vi "Select.vi"(0 "Father":u8[](array[numeric]) format="0x%02x", 2 "Mother":u8[](array[numeric]) format="0x%02x", 3 "Target":u8[](array[numeric]) format="0x%02x") -> (1 "Runnerup":u8[](array[numeric]) format="0x%02x", 4 "Winner":u8[](array[numeric]) format="0x%02x")   [LabVIEW 2013]
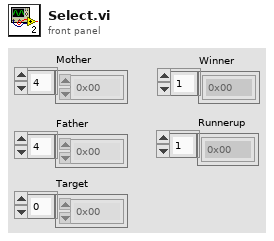
[diagram p1: front panel]
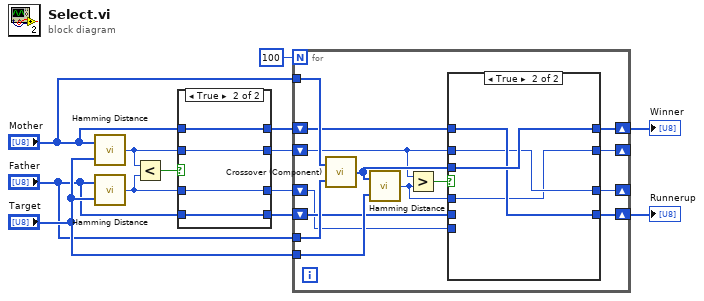
[diagram p0: block diagram]
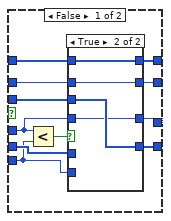
[diagram p2: hidden frame]
diagram:
  n1 = call "Hamming Distance.vi"("LED 2"="Target", "LED 1"="Mother") -> ("Hamming Distance"=w8:u32)
  n2 = call "Hamming Distance.vi"("LED 2"="Target", "LED 1"="Father") -> ("Hamming Distance"=w7:u32)
  n3 = Less?(x=w8, y=w7) -> (x < y?=w13:bool)
  n4 = case shown="True" w13 {
    tunnel: "Mother" -> [w16 w21]
    tunnel: "Father" -> [w17 w20]
    tunnel: [w17 w21] -> w12
    tunnel: [w16 w20] -> w11
    tunnel: w8 -> [w15 w19]
    tunnel: w7 -> [w14 w18]
    tunnel: [w14 w19] -> w6
    tunnel: [w15 w18] -> w5
    frame False {
    }
    frame True {
    }
  }
  n5 = for {
    N: 100 -> [_]
    shift-right: [w28] -> w10
    shift-left: w12 -> [w31]
    shift-right: [w25] -> w9
    shift-left: w11 -> [w29]
    tunnel: "Mother" -> [w35]
    tunnel: "Father" -> [w34]
    shift-right: [w27] -> _
    shift-left: w6 -> [w24]
    shift-right: [w26] -> _
    shift-left: w5 -> [w22]
    tunnel: "Target" -> [w33]
    n6 = call "Crossover (Component).vi"("Father"=w34, "Mother"=w35) -> ("Child"=w30:u8[])
    n7 = call "Hamming Distance.vi"("LED 2"=w33, "LED 1"=w30) -> ("Hamming Distance"=w23:u32)
    n8 = Greater?(x=w24, y=w23) -> (0:w32:bool)
    n9 = case shown="True" w32 {
      tunnel: w31 -> [w40 w57]
      tunnel: w30 -> [w45 w58]
      tunnel: w29 -> [w43 _]
      tunnel: [w41 w58] -> w28
      tunnel: [w39 w55] -> w27
      tunnel: [w36 w56] -> w26
      tunnel: [w37 w57] -> w25
      tunnel: w24 -> [w38 w56]
      tunnel: w23 -> [w44 w55]
      tunnel: w22 -> [w42 _]
      frame False {
        n10 = Less?(x=w44, y=w42) -> (x < y?=w46:bool)
        n11 = case shown="True" w46 {
          tunnel: w45 -> [_ w52]
          tunnel: w44 -> [_ w51]
          tunnel: w43 -> [w48 _]
          tunnel: w42 -> [w47 _]
          tunnel: [w50 w54] -> w41
          tunnel: w40 -> [w50 w54]
          tunnel: [w49 w53] -> w39
          tunnel: w38 -> [w49 w53]
          tunnel: [w48 w52] -> w37
          tunnel: [w47 w51] -> w36
          frame False {
          }
          frame True {
          }
        }
      }
      frame True {
      }
    }
  }
  "Winner" <- w10
  "Runnerup" <- w9
